vi "TCS_Rx.vi"() -> ()   [LabVIEW 2018]
uses:
  Stream/Stream.lvclass
  RxTx/RxTx.lvclass
  Stream/Stream.lvclass/Stream.ctl
panel:
  in  "RxTx in":refnum<class "RxTx.lvclass">
  in  "Stream in":refnum<class "Stream.lvclass">
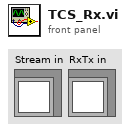
[diagram p1: front panel]
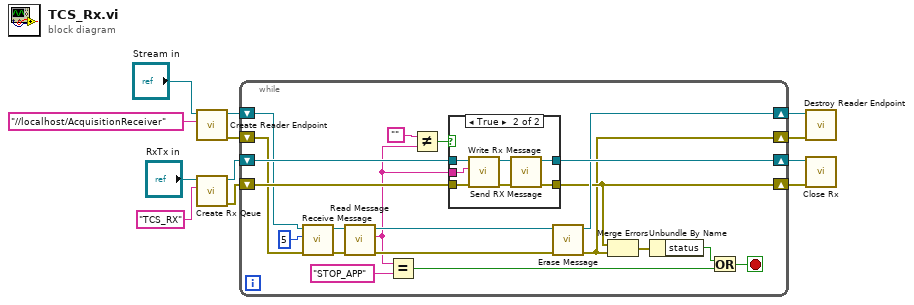
[diagram p0: block diagram]
diagram:
  n1 = call "Create Reader Endpoint.vi"("reader name"="//localhost/AcquisitionReceiver", "Stream in"="Stream in") -> ("error out"=w7:errorcluster, "Stream out"=w8:refnum<class "Stream.lvclass">)  [unwired: 8 in]
  n2 = call "Create Rx Qeue.vi"("Reader Name"="TCS_RX", "RxTx in"="RxTx in") -> ("error out"=w3:errorcluster, "RxTx out"=w4:refnum<class "RxTx.lvclass">)  [unwired: 8 in]
  n3 = while {
    shift-right: [w13] -> w11
    shift-left: w7 -> [w17]
    shift-right: [w23] -> w12
    shift-left: w8 -> [w18]
    shift-right: [w14] -> w5
    shift-left: w3 -> [w33]
    shift-right: [w31] -> w6
    shift-left: w4 -> [w32]
    stop <- w26 stop-if-true
    n4 = call "Receive Message.vi"("error in (no error)"=w17, "timeout ms"=5, "Stream in"=w18) -> ("error out"=w21:errorcluster, "Stream out"=w22:refnum<class "Stream.lvclass">)  [unwired: 7 in]
    n5 = call "Read Message.vi"("error in (no error)"=w21, "Stream in"=w22) -> ("error out"=w19:errorcluster, "Message"=w15:string, "Stream out"=w20:refnum<class "Stream.lvclass">)  [unwired: 7 in]
    n6 = Equal?(x=w15, y="STOP_APP" ("reader name")) -> (x = y?=w24:bool)
    n7 = Not Equal?(x="", y=w15) -> (x != y?=w28:bool)
    n8 = case shown="True" w28 {
      tunnel: w33 -> [w34 w38]
      tunnel: w32 -> [w35 w37]
      tunnel: [w35 w42] -> w31
      tunnel: [w34 w41] -> w14
      tunnel: w15 -> [_ w36]
      frame False {
      }
      frame True {
        n9 = call "Write Rx Message.vi"("error in (no error)"=w38, "Rx message"=w36, "RxTx in"=w37) -> ("error out"=w39:errorcluster, "RxTx out"=w40:refnum<class "RxTx.lvclass">)  [unwired: 7 in]
        n10 = call "Send RX Message.vi"("error in (no error)"=w39, "RxTx in"=w40) -> ("error out"=w41:errorcluster, "RxTx out"=w42:refnum<class "RxTx.lvclass">)  [unwired: 8 in]
      }
    }
    n11 = call "Erase Message.vi"("error in (no error)"=w19, "Stream in"=w20) -> ("error out"=w13:errorcluster, "Stream out"=w23:refnum<class "Stream.lvclass">)  [unwired: 8 in]
    n12 = Merge Errors(w14, w13) -> (w30:errorcluster)
    n13 = Unbundle By Name(w30) -> ("status"=w25:bool)
    n14 = Or(x=w25, y=w24) -> (x .or. y?=w26:bool)
  }
  n15 = call "Destroy Reader Endpoint.vi"("error in (no error)"=w11, "Stream in"=w12) -> ()  [unwired: 8 in, 2 out]
  n16 = call "Close Rx.vi"("error in (no error)"=w5, "RxTx in"=w6) -> ()  [unwired: 8 in, 2 out]
